vi "Error - Log Error.vi"(8 "error in (no error)":errorcluster, 11 "Error Data":T1) -> (0 "error out":errorcluster)   [LabVIEW 2017]
doc: "Generates (Open/Create) Log File and store all Error data\n[Covers: EH2]"
uses:
  Controls/Error Data.ctl
  Controls/Error Type.ctl
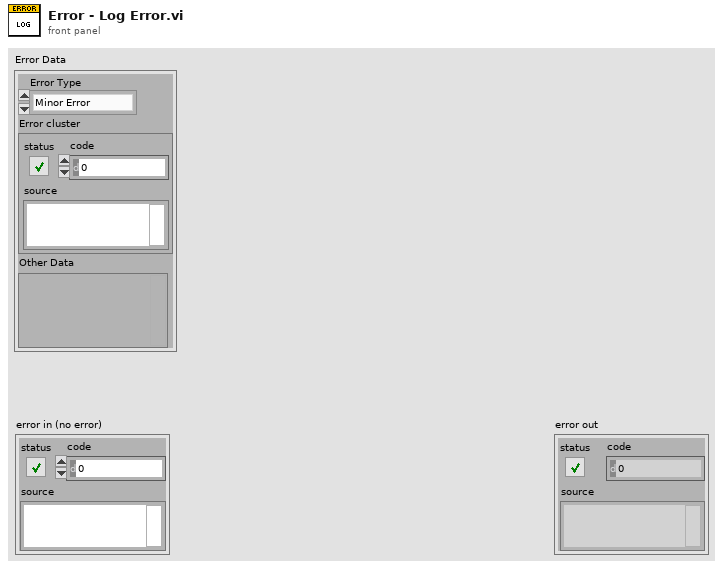
[diagram p1: front panel]
types:
  T1 = typedef "Error Data.ctl" = cluster{"Error Type":T2, "Error cluster":errorcluster, "Other Data":variant}
  T2 = typedef "Error Type.ctl" = enum16{"Minor Error", "Wash Cycle Error", "System Error", "Other Error"}
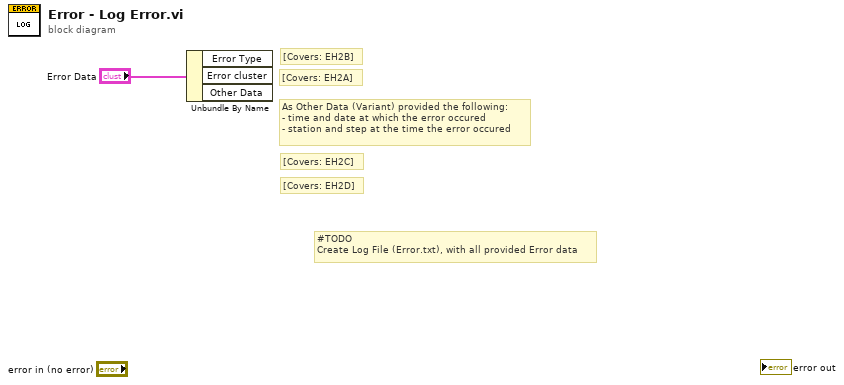
[diagram p0: block diagram]
diagram:
  # "#TODO\nCreate Log File (Error.txt), with all provided Error data"
  # "[Covers: EH2A]"
  # "[Covers: EH2B]"
  # "[Covers: EH2D]"
  # "[Covers: EH2C]"
  # "As Other Data (Variant) provided the following:\n- time and date at which the error occured\n- station and step at the time the error occured"
  n1 = Unbundle By Name("Error Data") -> ()  [unwired: 3 out]
